vi "SETKTVdll.vi"(8 "error in (no error)":errorcluster, 11 "Inputs":T2) -> (0 "error out":errorcluster, 3 "Outputs":T1)   [LabVIEW 2016]
doc: "subroutine SETKTVdll(icomp, jcomp, hmodij, fij, hfmix, ierr, herr, hmodij_length, hfmix_length, herr_length)\n\nSet mixture model and/or parameters.\n\nThis subroutine must be called after SETUP, but before any call to SETREF (for cases where energy, enthalpy,\nentropy, Gibbs energy, or the Helmholtz energy are required); it need not be called at all if the default mixture\nparameters (those read in by SETUP) are to be used. The component numbers icomp and jcomp must match\nthe order that is found in the hmx.bnc file for each binary pair, or, in the case where no interaction parameters\nare available in the hmx.bnc file, icomp and jcomp must be in the same order as was used in the call to SETUP.\nIf the numbers in these two integers are backwards, an error number and message will be returned, and nothing\nwill be changed. In this situation, switch the numbers and call this routine again.\n\nINPUTS:\nicomp -- Component i\njcomp -- Component j\nhmodij -- Mixing rule for the binary pair i,j (character*3)\n e.g. 'LJ1' (Lemmon-Jacobsen model)\n 'LM1' (modified Lemmon-Jacobsen model) or\n 'LIN' (linear mixing rules)\n 'KW0' (Wagner model)\n ‘RST’ Reset all pairs to values from original call to SETUP (all other inputs are ignored)\nfij -- Binary mixture parameters (array of dimension nmxpar; currently nmxpar is set to 6) The parameters will vary \n depending on hmodij. \n\n Kunz-Wagner model (KW0): \n fij(1) = betaT\n fij(2) = gammaT \n fij(3) = betaV \n fij(4) = gammaV\n fij(5) = Fpq \n fij(6) = ‘not used’\n\n Lemmon-Jacobsen model (LJ6):\n fij(1) = zeta \n fij(2) = xi \n fij(3) = Fpq \n fij(4) = beta\n fij(5) = gamma\n fij(6) = ‘not used’ \n\nhfmix -- File name (character*255) containing generalized parameters for the binary mixture model; this will usually \n be the same as the corresponding input to SETUP (e.g.,’hmx.bnc’)\n\nOUTPUTS:\nierr -- Error flag: 0 - Successful \n 111 - Error in opening mixture file \n -113 - Illegal i,j specification (i=j or i>nc or j>nc) \n 115 - Order of fluids is backwards from that in HMX.BNC\nherr -- Error string (character*255)\nhmodij_length -- length of variable hmodij (default: 3)\nhfmix_length -- length of variable hfmix (default: 255)\nherr_length -- length of variable herr (default: 255)"
uses:
  REFPROP.DLL
panel:
  # "REFPROP-SETKTVdll.vi"
  # "void  SETKTVdll(int32_t *icomp, int32_t *jcomp, CStr hmodij, double *fij, CStr hfmix, int32_t ierr, CStr herr, int32_t hmodj_length, int32_t hfmix_length, int32_t herr_length)"
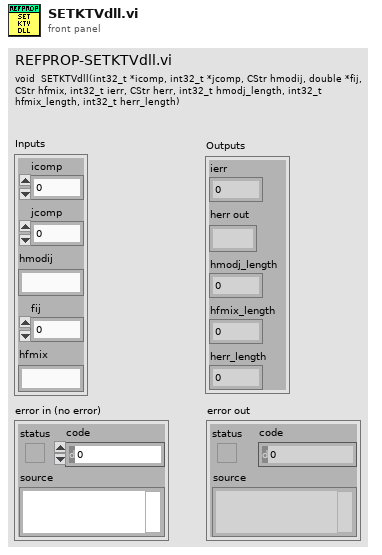
[diagram p1: front panel]
types:
  T1 = cluster{"ierr":i32, "herr out":string, "hmodj_length":i32, "hfmix_length":i32, "herr_length":i32}
  T2 = cluster{"icomp":i32, "jcomp":i32, "hmodij":string, "fij":dbl, "hfmix":string}
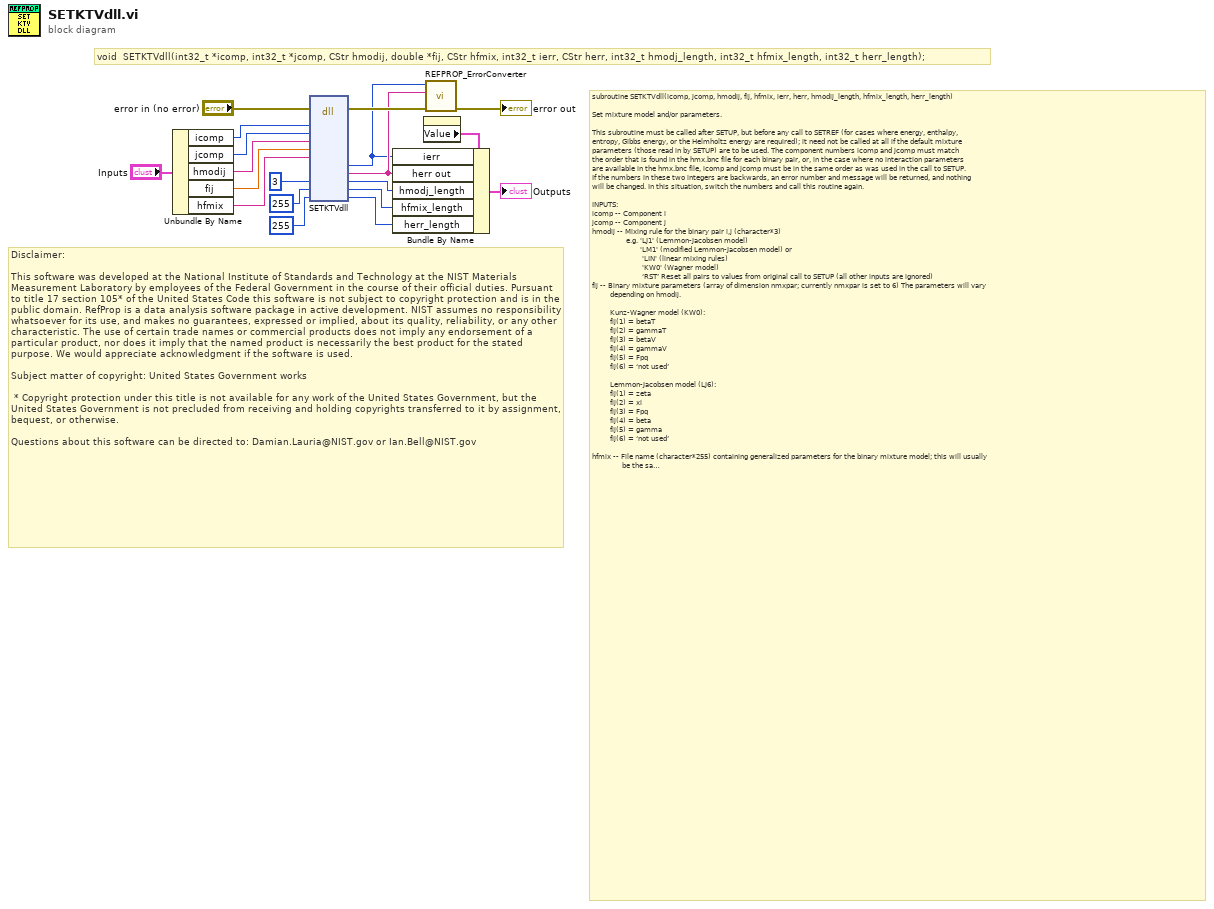
[diagram p0: block diagram]
diagram:
  # "Disclaimer:\n\nThis software was developed at the National Institute of Standards and Technology at the NIST Materials Measurement Laboratory by employees of the Federal Government in the course of their official duties. Pursuant to title 17 section 105* of the United States Code this software is not subject to copyright protection and is in the public domain. RefProp is a data analysis software package in active development. NIST assumes no responsibility whatsoever for its use, and makes no guarantees, expressed or implied, about its quality, reliability, or any other characteristic. The use of certain trade names or commercial products does not imply any endorsement of a particular product, nor does it imply that the named product is necessarily the best product for the stated purpose. We would appreciate acknowledgment if the software is used.\n \nSubject matter of copyright: United States Government works\n  \n * Copyright protection under this title is not available for any work of the United States Government, but the United States Government is not precluded from receiving and holding copyrights transferred to it by assignment, bequest, or otherwise.\n\nQuestions about this software can be directed to: Damian.Lauria@NIST.gov or Ian.Bell@NIST.gov"
  # "void  SETKTVdll(int32_t *icomp, int32_t *jcomp, CStr hmodij, double *fij, CStr hfmix, int32_t ierr, CStr herr, int32_t hmodj_length, int32_t hfmix_length, int32_t herr_length);"
  # "subroutine SETKTVdll(icomp, jcomp, hmodij, fij, hfmix, ierr, herr, hmodij_length, hfmix_length, herr_length)\n\nSet mixture model and/or parameters.\n\nThis subroutine must be called after SETUP, but before any call to SETREF (for cases where energy, enthalpy,\nentropy, Gibbs energy, or the Helmholtz energy are required); it need not be called at all if the default mixture\nparameters (those read in by SETUP) are to be used. The component numbers icomp and jcomp must match\nthe order that is found in the hmx.bnc file for each binary pair, or, in the case where no interaction parameters\nare available in the hmx.bnc file, icomp and jcomp must be in the same order as was used in the call to SETUP.\nIf the numbers in these two integers are backwards, an error number and message will be returned, and nothing\nwill be changed. In this situation, switch the numbers and call this routine again.\n\nINPUTS:\nicomp -- Component i\njcomp -- Component j\nhmodij -- Mixing rule for the binary pair i,j (character*3)\n                 e.g. 'LJ1' (Lemmon-Jacobsen model)\n                        'LM1' (modified Lemmon-Jacobsen model) or\n                         'LIN' (linear mixing rules)\n                         'KW0' (Wagner model)\n                         ‘RST’ Reset all pairs to values from original call to SETUP (all other inputs are ignored)\nfij -- Binary mixture parameters (array of dimension nmxpar; currently nmxpar is set to 6) The parameters will vary \n         depending on hmodij. \n\n         Kunz-Wagner model (KW0):  \n         fij(1) = betaT\n         fij(2) = gammaT \n         fij(3) = betaV \n         fij(4) = gammaV\n         fij(5) = Fpq \n         fij(6) = ‘not used’\n\n         Lemmon-Jacobsen model (LJ6):\n         fij(1) = zeta \n         fij(2) = xi \n         fij(3) = Fpq \n         fij(4) = beta\n         fij(5) = gamma\n         fij(6) = ‘not used’ \n\nhfmix -- File name (character*255) containing generalized parameters for the binary mixture model; this will usually \n               be the same as the corresponding input to SETUP (e.g.,’hmx.bnc’)\n\nOUTPUTS:\nierr -- Error flag: 0 - Successful \n                             111 - Error in opening mixture file \n                           -113 - Illegal i,j specification (i=j or i>nc or j>nc) \n                             115 - Order of fluids is backwards from that in HMX.BNC\nherr -- Error string (character*255)\nhmodij_length -- length of variable hmodij (default: 3)\nhfmix_length -- length of variable hfmix (default: 255)\nherr_length -- length of variable herr (default: 255)"
  n1 = Unbundle By Name("Inputs") -> ("icomp"=w12:i32, "jcomp"=w11:i32, "hmodij"=w10:string, "fij"=w9:dbl, "hfmix"=w8:string)
  n2 = dll-call lib="S:/009 - Testing/02 - Performance Testing/REFPROP/REFPROP.*" fn="SETKTVdll"(error in="error in (no error)", "icomp"=w12, "jcomp"=w11, "hmodij"=w10, "fij"=w9, "hfmix"=w8, "hmodj_length"=3 ("hfmix_length"), "hfmix_length"=255, "herr_length"=255 ("hfmix_length")) -> (error out=w19:errorcluster, "ierr"=w1:i32, "herr"=w2:string, "hmodj_length"=w6:i32, "hfmix_length"=w5:i32, "herr_length"=w4:i32)  [unwired: 10 in, 1 out]
  n3 = property on="Outputs" class="Clust (strict)"() -> ("Value"=w7:T1)  [unwired: 2 in, 2 out]
  n4 = Bundle By Name(cluster=w7, "ierr"=w1, "herr out"=w2, "hmodj_length"=w6, "hfmix_length"=w5, "herr_length"=w4) -> (→"Outputs":T1)
  n5 = call "REFPROP_ErrorConverter.vi"("error in (no error)"=w19, "Error Message"=w2, "Error Code"=w1) -> ("error out"=→"error out":errorcluster)  [unwired: 8 in]
